vi "Sign In.vi"(0 "ICanCommunicate In":refnum<class "Process.lvclass">, 7 "Message Handler":refnum<class "ICanCommunicate.lvclass">, 11 "Error In":errorcluster) -> (4 "ICanCommunicate Out":refnum<class "Process.lvclass">, 15 "Error Out":errorcluster)   [LabVIEW 2023, in "Process.lvclass"]
uses:
  Process.lvclass
  H:/Desktop/LabVIEW/LabView Repo/Framework/Interfaces/ICanCommunicate/ICanCommunicate.lvclass
  Interfaces/ICanCommunicate/ICanCommunicate.lvclass
  Subclasses/Message Handler/Message Handler.lvclass
  Interfaces/ICanCommunicate/Process Refs.ctl
  Interfaces/ICanCommunicate/ToProcessQueue.ctl
  Interfaces/ICanCommunicate/Message.ctl
  Interfaces/ICanCommunicate/FromProcessQueue.ctl
  Interfaces/ICanCommunicate/ProcessSyncQueue.ctl
  Process.lvclass/Process.ctl
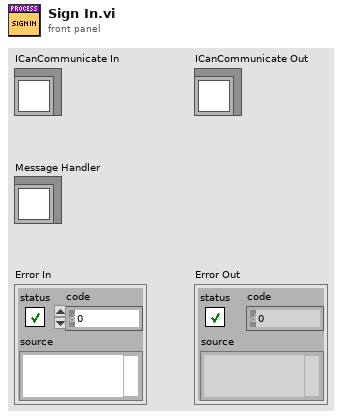
[diagram p1: front panel]
types:
  T1 = typedef "ICanCommunicate.lvclass/Process Refs.ctl" = cluster{"ToProcessQueue":T2, "FromProcessQueue":T3, "ProcessSyncQueue":T4, "ProcessViRef":refnum<vi>}
  T2 = typedef "ICanCommunicate.lvclass/ToProcessQueue.ctl" = refnum<queue>
  T3 = typedef "ICanCommunicate.lvclass/FromProcessQueue.ctl" = refnum<queue>
  T4 = typedef "ICanCommunicate.lvclass/ProcessSyncQueue.ctl" = refnum<queue>
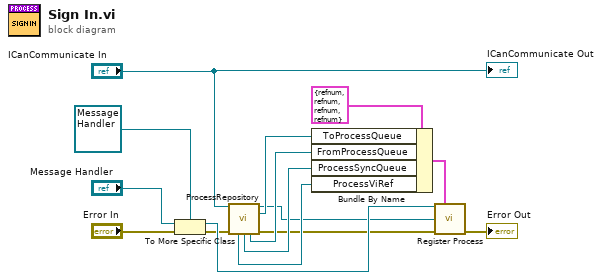
[diagram p0: block diagram]
diagram:
  n1 = To More Specific Class(target class=refnum<class "Message Handler.lvclass"> refnum ("Process"), reference="Message Handler", error in="Error In") -> (specific class reference=w13:refnum<class "Message Handler.lvclass">, error out=w9:errorcluster)
  n2 = call-dynamic "ProcessRepository.vi"("Process In"="ICanCommunicate In", "Error In"=w9) -> ("Process Out"=w1:refnum<class "Process.lvclass">, "ToProcessQueue"=w7:T2, "ProcessViRef"=w4:refnum<vi>, "ProcessSyncQueue"=w5:T4, "FromProcessQueue"=w6:T3, "Error Out"=w2:errorcluster)  [unwired: 7 in, 1 out]
  n3 = Bundle By Name(cluster=T1 {"ToProcessQueue"=refnum, "FromProcessQueue"=refnum, "ProcessSyncQueue"=refnum, "ProcessViRef"=refnum} ("ProcessRefs"), "ToProcessQueue"=w7, "FromProcessQueue"=w6, "ProcessSyncQueue"=w5, "ProcessViRef"=w4) -> (w3:T1)
  n4 = call-dynamic "Register Process.vi"("Message Handler In"=w13, "ProcessRefs"=w3, "Process"=w1, "Error In"=w2) -> ("Error Out"=→"Error Out":errorcluster)  [unwired: 10 in, 1 out]
  "ICanCommunicate Out" <- "ICanCommunicate In"
